vi "thorlabs_panel_register_events.vi"(8 "error in (no error)":errorcluster, 11 "thorlabs_panel in":refnum<class "thorlabs_panel.lvclass">) -> (0 "error out":errorcluster, 2 "event_refs cluster":T1, 3 "thorlabs_panel out":refnum<class "thorlabs_panel.lvclass">)   [LabVIEW 2015, in "thorlabs_panel.lvclass"]
uses:
  thorlabs_panel.lvclass
  thorlabs_event_refs.ctl
  thorlabs_events.ctl
  thorlabs_panel.lvclass/thorlabs_panel.ctl
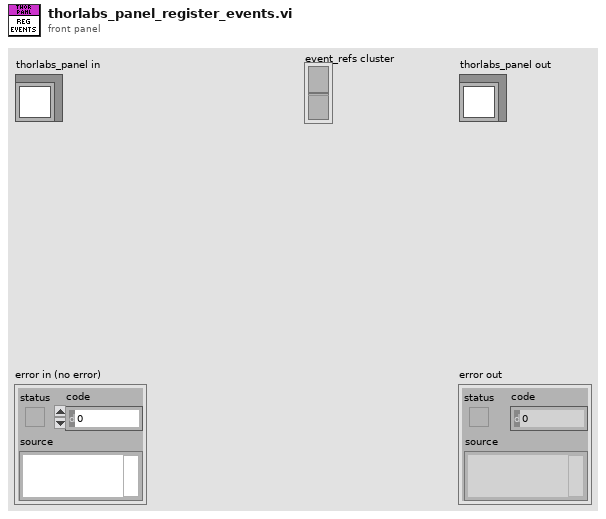
[diagram p1: front panel]
types:
  T1 = typedef "thorlabs_event_refs.ctl" = cluster{"Event Registration Refnum":refnum<event-registration>, "Event Registration Refnum":refnum<event-registration>}
  T2 = typedef "thorlabs_events.ctl" = cluster{"mcl_status":refnum<user-event>, "piezo_positions":refnum<user-event>}
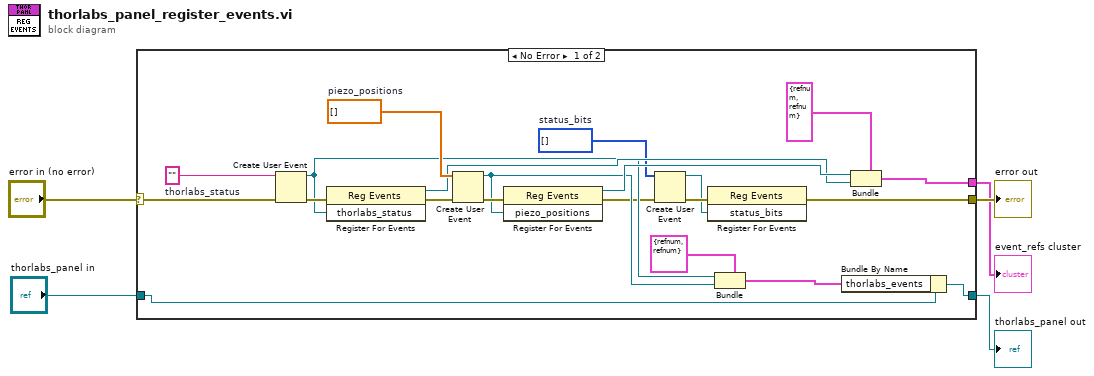
[diagram p0: block diagram]
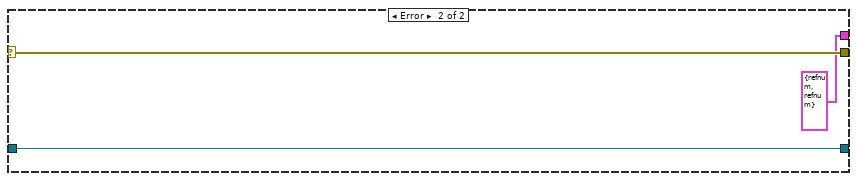
[diagram p2: hidden frame]
diagram:
  n1 = case shown="No Error" "error in (no error)" {
    selector: "error in (no error)" -> [w25 w29]
    tunnel: [w7 w29] -> w4
    tunnel: [w11 w28] -> w2
    tunnel: "thorlabs_panel in" -> [w13 w28]
    tunnel: [w14 T1 {"Event Registration Refnum"=refnum, "Event Registration Refnum"=refnum} ("output cluster")] -> w1
    frame No Error {
      w9 = i32[] []  # status_bits
      w21 = dbl[] []  # piezo_positions
      w26 = ""  # thorlabs_status
      n2 = Create User Event(user event datatype=w26, error in=w25) -> (user event=w18:refnum<user-event>, error out=w24:errorcluster)
      n3 = register-events(error in=w24, w18) -> (reference out=w19:refnum<event-registration>, error out=w22:errorcluster)  [unwired: 1 in]
      n4 = Create User Event(user event datatype=w21, error in=w22) -> (user event=w17:refnum<user-event>, error out=w23:errorcluster)
      n5 = register-events(error in=w23, w17) -> (reference out=w20:refnum<event-registration>, error out=w10:errorcluster)  [unwired: 1 in]
      n6 = Create User Event(user event datatype=w9, error in=w10) -> (user event=w6:refnum<user-event>, error out=w8:errorcluster)
      n7 = register-events(error in=w8, w6) -> (error out=w7:errorcluster)  [unwired: 1 in, 1 out]
      n8 = Bundle(cluster=T2 {"mcl_status"=refnum, "piezo_positions"=refnum} ("output cluster"), "mcl_status"=w18, "piezo_positions"=w17) -> (w12:T2)
      n9 = Bundle By Name(cluster=w13, "thorlabs_events"=w12) -> (w11:refnum<class "thorlabs_panel.lvclass">)
      n10 = Bundle(cluster=T1 {"Event Registration Refnum"=refnum, "Event Registration Refnum"=refnum} ("output cluster"), "Event Registration Refnum"=w20, "Event Registration Refnum"=w19) -> (w14:T1)
    }
    frame Error {
    }
  }
  "error out" <- w4
  "thorlabs_panel out" <- w2
  "event_refs cluster" <- w1
